vi "反馈节点 与 移位寄存器.vi"() -> ()   [LabVIEW 2023]
panel:
  out "Numeric 2":i32
  out "Array 3":i32[][](array[numeric])
  out "Numeric":i32
  out "Array 2":i32[][](array[numeric])
  out "Array":i32[][](array[numeric])
  out "x+y":i32
  # "反馈节点 与 移位寄存器"
  # "这个例子 示范的是  反馈节点 与移位寄存器  的 共同点"
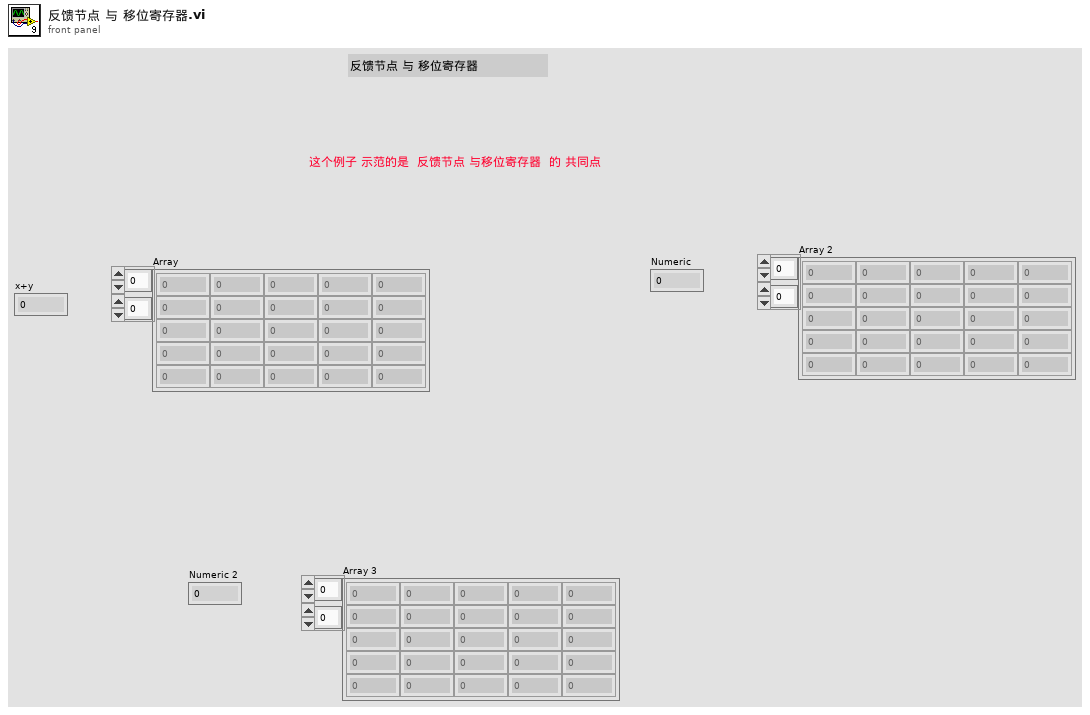
[diagram p1: front panel]
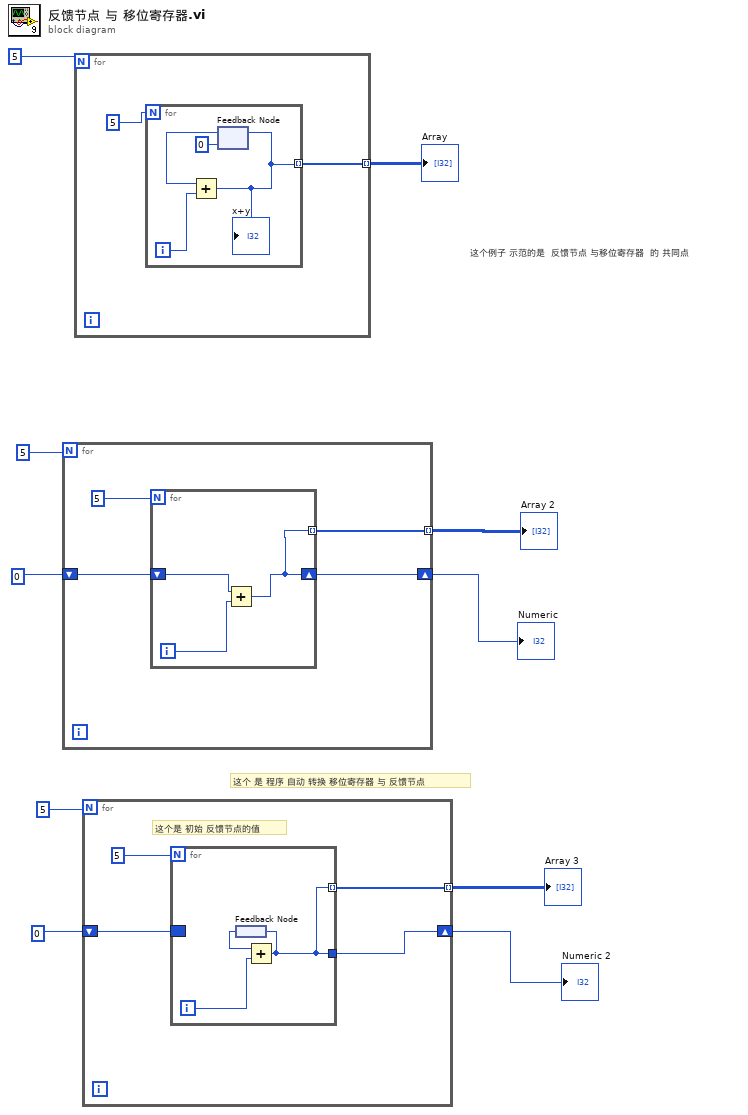
[diagram p0: block diagram]
diagram:
  # "这个 是 程序 自动 转换 移位寄存器 与 反馈节点"
  # "这个例子 示范的是  反馈节点 与移位寄存器  的 共同点"
  n1 = for {
    N: 5 -> [_]
    shift-right: [w11] -> w5
    shift-left: 0 -> [w13]
    tunnel: [w12] -> w6 mode=indexing
    n2 = for {
      N: 5 -> [_]
      shift-right: [w15] -> w11
      shift-left: w13 -> [w17]
      tunnel: [w15] -> w12 mode=indexing
      i -> [w16]
      n3 = Add(x=w17, y=w16) -> (x+y=w15:i32)
    }
  }
  "Array 2" <- w6
  "Numeric" <- w5
  n4 = for {
    N: 5 -> [_]
    tunnel: [w18] -> w9 mode=indexing
    n5 = for {
      N: 5 -> [_]
      tunnel: [w20] -> w18 mode=indexing
      i -> [w23]
      n6 = feedback #1(0) -> (w22:i32)
      n7 = Add(x=w22, y=w23) -> (x+y=w20:i32)
      "x+y" <- w20
      n8 = feedback-in #1(w20) -> ()
    }
  }
  "Array" <- w9
  n9 = for {
    N: 5 -> [_]
    shift-right: [w24] -> w1
    shift-left: 0 -> [w26]
    tunnel: [w25] -> w2 mode=indexing
    # "这个是 初始 反馈节点的值"
    n10 = for {
      N: 5 -> [_]
      tunnel: [w28] -> w25 mode=indexing
      border: w26 -> [_]
      tunnel: [w28] -> w24
      i -> [w29]
      n11 = feedback #2() -> (w30:i32)
      n12 = Add(x=w30, y=w29) -> (x+y=w28:i32)
      n13 = feedback-in #2(w28) -> ()
    }
  }
  "Array 3" <- w2
  "Numeric 2" <- w1
